vi "tip_light_error_test.vi"() -> (0 "Tip residues":dbl[][](array[numeric]) format="%#.0f", 3 "Tip RMS":dbl format="%#.0f")   [LabVIEW 2014]
uses:
  <vilib>/Analysis/Matrix/Datatypes/RealMatrix.ctl
  asap/labview/testing/calibration_task.ctl
  <vilib>/Analysis/Matrix/Numeric/Conversions/Array To Matrix - RA2.vi
  <vilib>/Analysis/Matrix/NI_Matrix.lvlib
panel:
  in  "z offset":sgl=3000.0
  out "Handle pose":T1
  out "Handle lights":sgl[][](array[numeric]) format="%#.0f"
  out "Tip pose":T1
  out "Tip lights":sgl[][](array[numeric]) format="%#.0f"
  out "Handle residues":dbl[][](array[numeric]) format="%#.0f"
  out "Handle RMS":dbl format="%#.0f"
  in  "Test mode":bool
  in  "XYZ in":sgl[][](array[numeric])=[[7519.664, 4298.2593, 2461.168], [-946.79065, 2755.9197, 13726.396], [-7865.031, 4979.443, 1497.3561], [627.65344, 4790.8125, -13265.299], [1659.564, 3313.333, -4070.8655], [4632.295, 4763.3896, -13001.61]] format="%#.2f"
  # "This is a mutated version of tip_light_error which can be used to test the light initialization and pose solution for consistency."
  # "Run with \"Test mode\" off and with \"micron_ui\" running, set \"Test mode\" to on, then stop micron_ui. This saves the light positions in \"XYZ in\". Then you can run and debug the pose solution VIs without completely bogging down the realtime loop."
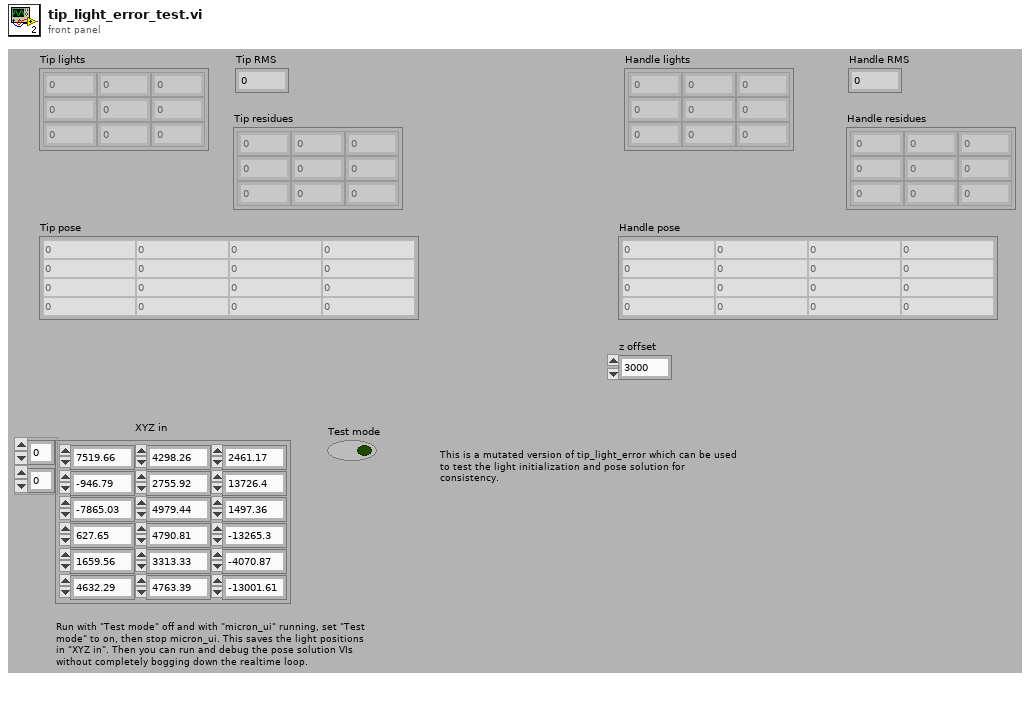
[diagram p1: front panel]
types:
  T1 = typedef "NI_Matrix.lvlib/RealMatrix.ctl" = dbl[][]
  T2 = typedef "calibration_task.ctl" = enum16{"Tip offset", "RCM offset", "Tip lights", "Handle lights"}
  T3 = typedef "probe_calibration.ctl" = sgl[][]
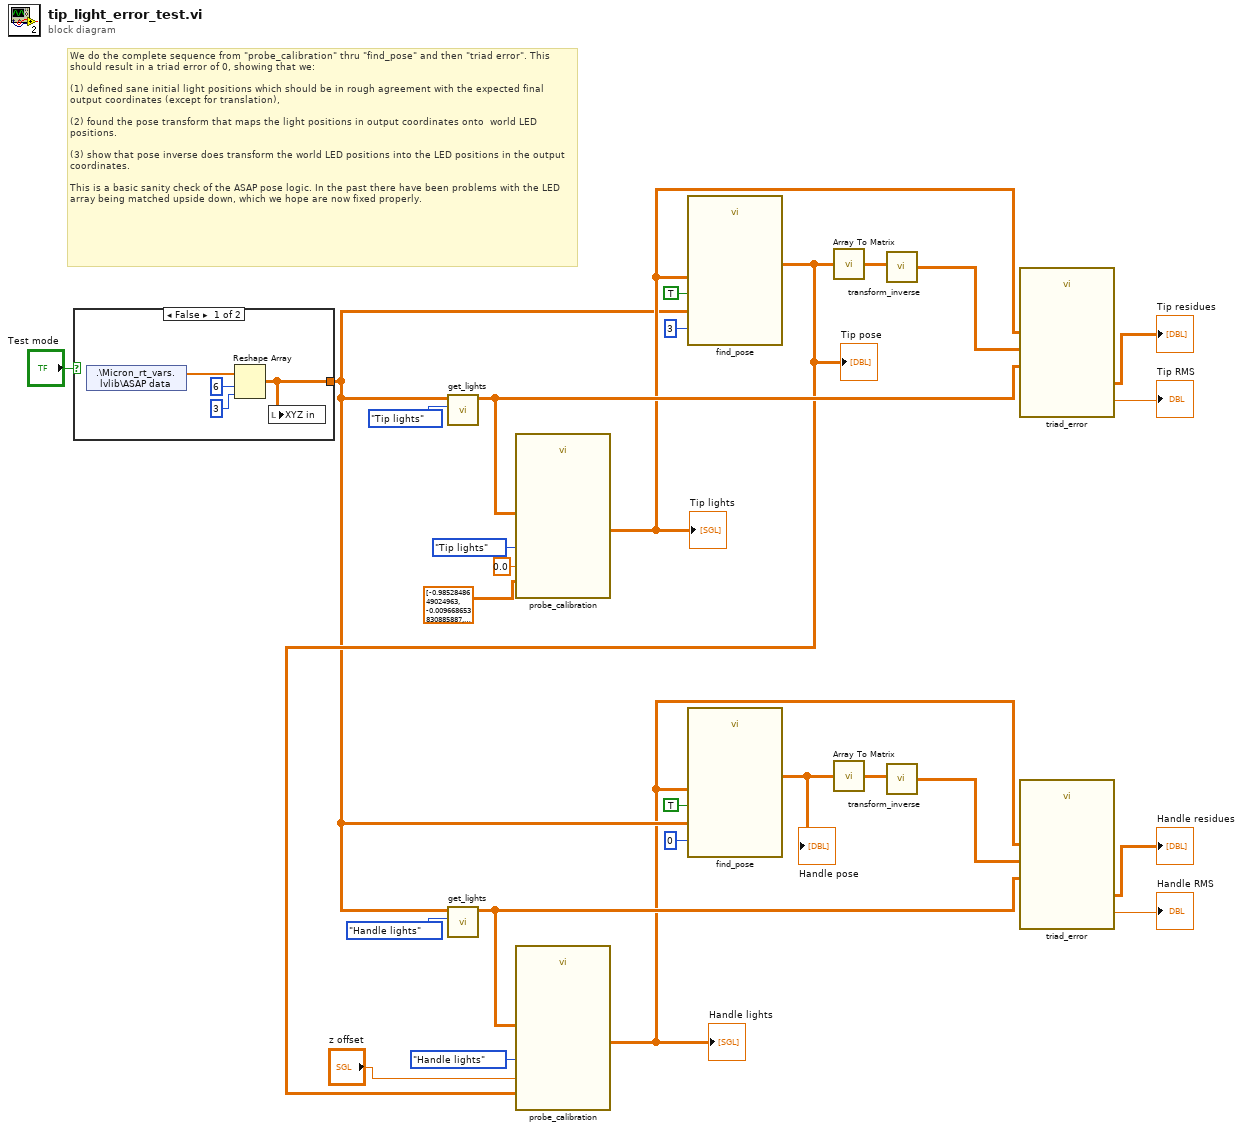
[diagram p0: block diagram]
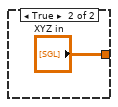
[diagram p2: hidden frame]
diagram:
  # "We do the complete sequence from \"probe_calibration\" thru \"find_pose\" and then \"triad error\". This should result in a triad error of 0, showing that we:\n\n(1) defined sane initial light positions which should be in rough agreement with the expected final output coordinates (except for translation), \n\n(2) found the pose transform that maps the light positions in output coordinates onto  world LED positions.\n\n(3) show that pose inverse does transform the world LED positions into the LED positions in the output coordinates.\n\nThis is a basic sanity check of the ASAP pose logic. In the past there have been problems with the LED array being matched upside down, which we hope are now fixed properly."
  n1 = case shown="False" "Test mode" {
    tunnel: [w28 "XYZ in"] -> w4
    frame False {
      n2 = shared-variable ".\\Micron_rt_vars.lvlib\\ASAP data"() -> (w29:sgl[])  [unwired: 2 out]
      n3 = Reshape Array(w29, 6 ("dimension size"), 3 ("dimension size")) -> (w28:sgl[][])
      n4 = local write "XYZ in"(w28) -> ()
    }
    frame True {
    }
  }
  n5 = call "get_lights.vi"("Selector"=enum16{"Handle lights", "Tip lights"}."Tip lights", "ASAP data"=w4) -> ("Light positions"=w16:T3)  [unwired: 9 in]
  n6 = call "get_lights.vi"("Selector"=enum16{"Handle lights", "Tip lights"}."Handle lights", "ASAP data"=w4) -> ("Light positions"=w15:T3)  [unwired: 9 in]
  n7 = call "probe_calibration.vi"("z offset"=sgl 0.0, "Calibration task"=calibration_task."Tip lights", "World light positions"=w16, "Output pose"=dbl[][] [[-0.9852848649024963, -0.009668653830885887, 0.17064659297466278, 1828.239501953125], [0.020961355417966843, 0.9840268492698669, 0.17678126692771912, 5689.6396484375], [-0.16963009536266327, 0.1777568906545639, -0.9693441987037659, -8739.658203125], [0.0, 0.0, 0.0, 1.0]]) -> ("Probe calibration"=w5:T3)  [unwired: 7 out]
  "Tip lights" <- w5
  n8 = call "find_pose.vi"("Position valid"=TRUE, "Light positions"=w5, "XYZ index"=3, "XYZ in"=w4) -> ("Pose"=w6:T1)  [unwired: 1 in, 6 out]
  "Tip pose" <- w6
  n9 = call "probe_calibration.vi"("z offset"="z offset", "Calibration task"=calibration_task."Handle lights", "World light positions"=w15, "Output pose"=w6) -> ("Probe calibration"=w3:T3)  [unwired: 7 out]
  "Handle lights" <- w3
  n10 = call "find_pose.vi"("Position valid"=TRUE, "Light positions"=w3, "XYZ index"=0, "XYZ in"=w4) -> ("Pose"=w2:T1)  [unwired: 1 in, 6 out]
  "Handle pose" <- w2
  n11 = call-poly <vilib>:"Array To Matrix.vi"("Real 2D Array"=w6) -> ("Real Matrix"=w24:T1)
  n12 = call-poly <vilib>:"Array To Matrix.vi"("Real 2D Array"=w2) -> ("Real Matrix"=w9:T1)
  n13 = call "transform_inverse.vi"("Transform"=w24) -> ("Inverse transform"=w23:T1)
  n14 = call "transform_inverse.vi"("Transform"=w9) -> ("Inverse transform"=w10:T1)
  n15 = call "triad_error.vi"("Measured positions"=w16, "Measure transform"=w23, "Calibrated positions"=w5) -> ("Residues"=→"Tip residues":T3, "RMS error"=→"Tip RMS":dbl)  [unwired: 7 in]
  n16 = call "triad_error.vi"("Measured positions"=w15, "Measure transform"=w10, "Calibrated positions"=w3) -> ("Residues"=→"Handle residues":T3, "RMS error"=→"Handle RMS":dbl)  [unwired: 7 in]
